vi "Create Queue.vi"(8 "Error In":errorcluster, 11 "Queue Name (Optional)":string) -> (0 "Error Out":errorcluster, 3 "Queue Ref":refnum<queue>)   [LabVIEW 2014, in "SLL QSM.lvlib"]
doc: "Create Queue Reference based on the VI instance name."
uses:
  SLL QSM.lvlib
  Typedefs/Queue Type.ctl
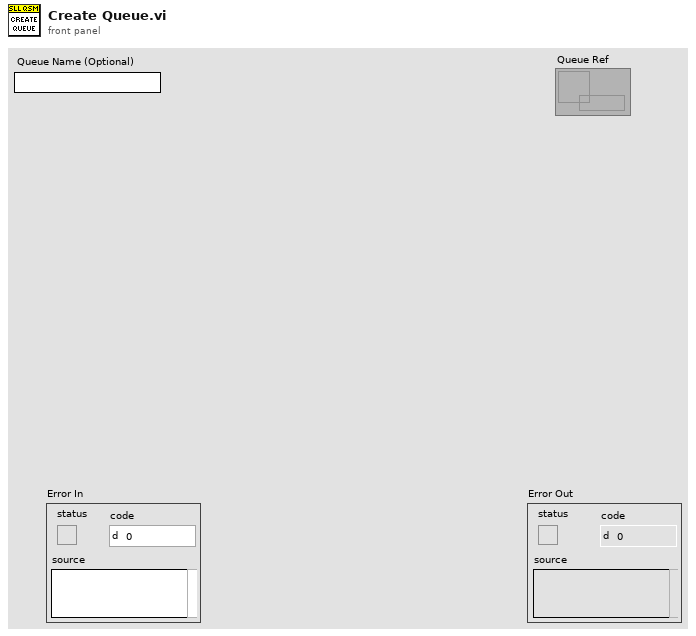
[diagram p1: front panel]
types:
  T1 = typedef "SLL QSM.lvlib/Queue Type.ctl" = cluster{"State":string, "Data":variant}
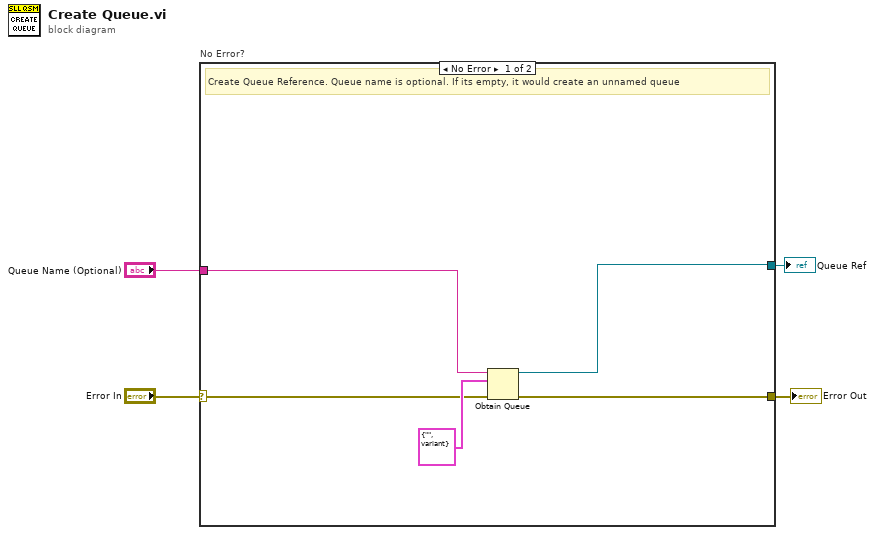
[diagram p0: block diagram]
diagram:
  n1 = case "No Error?" shown="No Error" "Error In" {
    selector: "Error In" -> [w8 w10]
    tunnel: [w7 w10] -> w4
    tunnel: [w6 _] -> w2
    tunnel: "Queue Name (Optional)" -> [w5 _]
    frame No Error {
      # "Create Queue Reference. Queue name is optional. If its empty, it would create an unnamed queue"
      n2 = Obtain Queue(name (unnamed)=w5, element data type=T1 {"State"="", "Data"=variant} ("Queue Type"), error in (no error)=w8) -> (queue out=w6:refnum<queue>, error out=w7:errorcluster)  [unwired: 2 in, 1 out]
    }
    frame Error {
    }
  }
  "Error Out" <- w4
  "Queue Ref" <- w2
